vi "Delay for Calibration.vi"(8 "Error In":errorcluster caption="Fehler (Eingang)", 10 "Delay (ms)":i32, 11 "Frame Name":string="Test") -> (0 "Error Out":errorcluster caption="Fehler (Ausgang)")   [LabVIEW 2017]
panel:
  out "Calibration in Progress ...":i32(slide) scale=0.0..300.0
  out "String":string
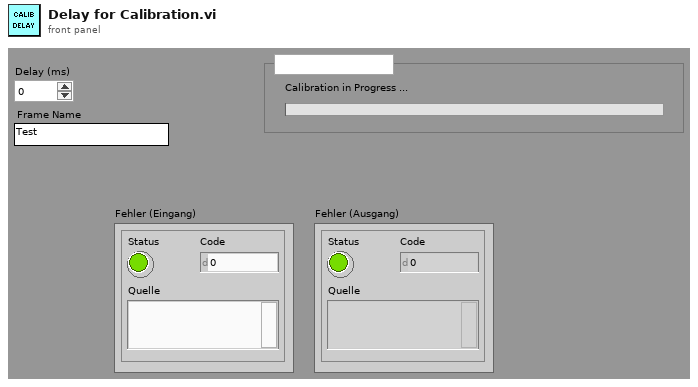
[diagram p1: front panel]
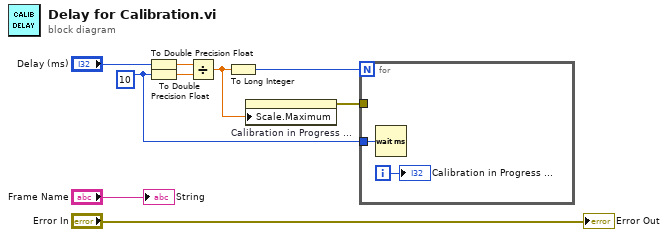
[diagram p0: block diagram]
diagram:
  w4 = u32 10 ("Zu wartende ms")
  n1 = To Double Precision Float(number="Delay (ms)") -> (double precision float=w7:dbl)
  n2 = To Double Precision Float(number=w4) -> (double precision float=w6:dbl)
  n3 = Divide(x=w7, y=w6) -> (x/y=w3:dbl)
  n4 = To Long Integer(number=w3) -> (32bit integer=w2:i32)
  n5 = property on="Calibration in Progress ..." class="Slide (strict)"("Scale.Maximum"=w3) -> (error out=w1:errorcluster)  [unwired: 2 in, 1 out]
  n6 = for {
    N: w2 -> [_]
    tunnel: w4 -> [w10]
    tunnel: w1 -> [_]
    i -> [w11]
    n7 = Wait (ms)(milliseconds to wait=w10) -> ()  [unwired: 1 out]
    "Calibration in Progress ..." <- w11
  }
  "String" <- "Frame Name"
  "Error Out" <- "Error In"
